vi "Read Lockin_Vsg.json.vi"(8 "error in (no error)":errorcluster, 10 "file (use dialog)":path, 11 "Transport in":refnum<class "SMO.Transport.lvclass">) -> (0 "error out":errorcluster, 2 "Lockin_Vsg":T1, 3 "Transport out":refnum<class "SMO.Transport.lvclass">)   [LabVIEW 2019, in "SMO.Transport.lvclass"]
uses:
  SMO.Transport.lvclass
  <vilib>/addons/_JKI.lib/Serialization/JSON/JKI JSON Serialization.lvlib
  Typedefs/Lockin_Vsg JSON--Cluster.ctl
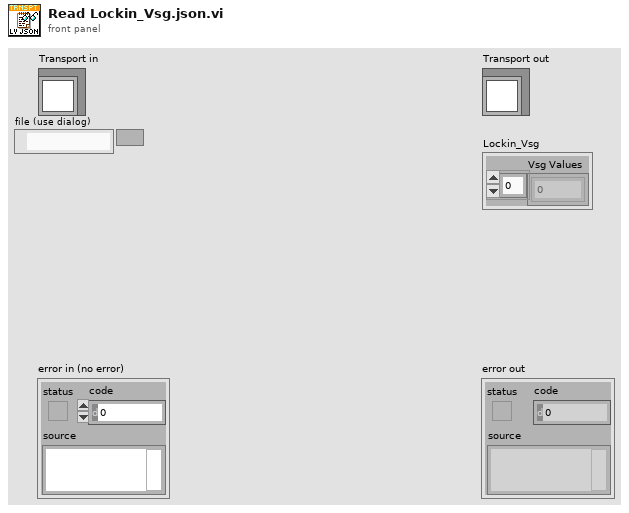
[diagram p1: front panel]
types:
  T1 = typedef "SMO.Transport.lvclass/Lockin_Vsg JSON--Cluster.ctl" = cluster{"Vsg Values":dbl[]}
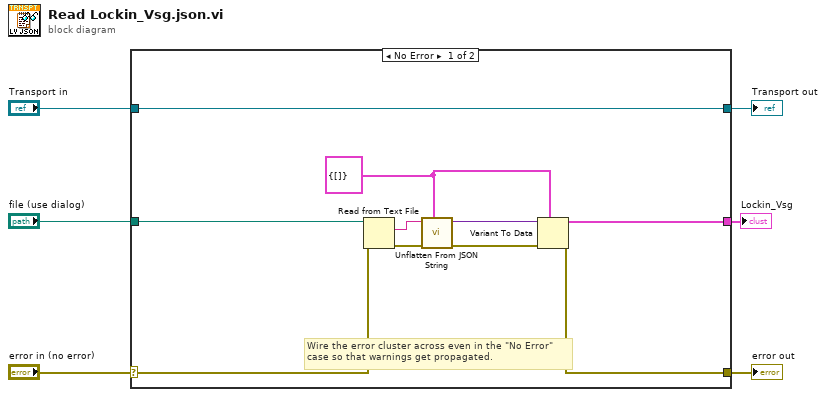
[diagram p0: block diagram]
diagram:
  n1 = case shown="No Error" "error in (no error)" {
    selector: "error in (no error)" -> [w9 w18]
    tunnel: [w8 w18] -> w5
    tunnel: [w16 w17] -> w3
    tunnel: "Transport in" -> [w16 w17]
    tunnel: [w11 _] -> w2
    tunnel: "file (use dialog)" -> [w10 _]
    frame No Error {
      w7 = T1 {"Vsg Values"=[]} ("Lockin_Vsg")
      # "Wire the error cluster across even in the \"No Error\"\ncase so that warnings get propagated."
      n2 = Read from Text File(file (use dialog)=w10, error in=w9) -> (text=w14:string, error out=w15:errorcluster)  [unwired: 2 in, 2 out]
      n3 = call <vilib>:"Unflatten From JSON String.vi"("Type and Defaults"=w7, "error in (no error)"=w15, "JSON String"=w14) -> ("error out"=w13:errorcluster, "Variant"=w12:variant)  [unwired: 7 in]
      n4 = Variant To Data(error in=w13, type=w7, Variant=w12) -> (data=w11:T1, error out=w8:errorcluster)
    }
    frame Error {
    }
  }
  "error out" <- w5
  "Transport out" <- w3
  "Lockin_Vsg" <- w2
